vi "Comm_relay_sw..vi"(8 "Error in":errorcluster, 9 "Columns":i32[](array[numeric]), 10 "Row":i32, 11 "instrument handle in":refnum<k15>) -> (0 "error out":errorcluster, 3 "instrument handle out":refnum<k15>)   [LabVIEW 2016]
uses:
  <instrlib>/niSwitch/niSwitch.LLB/niSwitch Connect Channels (Single).vi
  <instrlib>/niSwitch/niSwitch.LLB/niSwitch Disconnect Channels (Single).vi
panel:
  in  "number of columns":i32=16
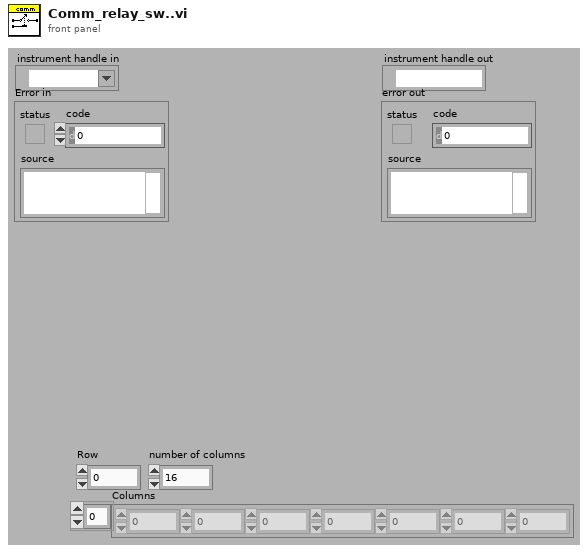
[diagram p1: front panel]
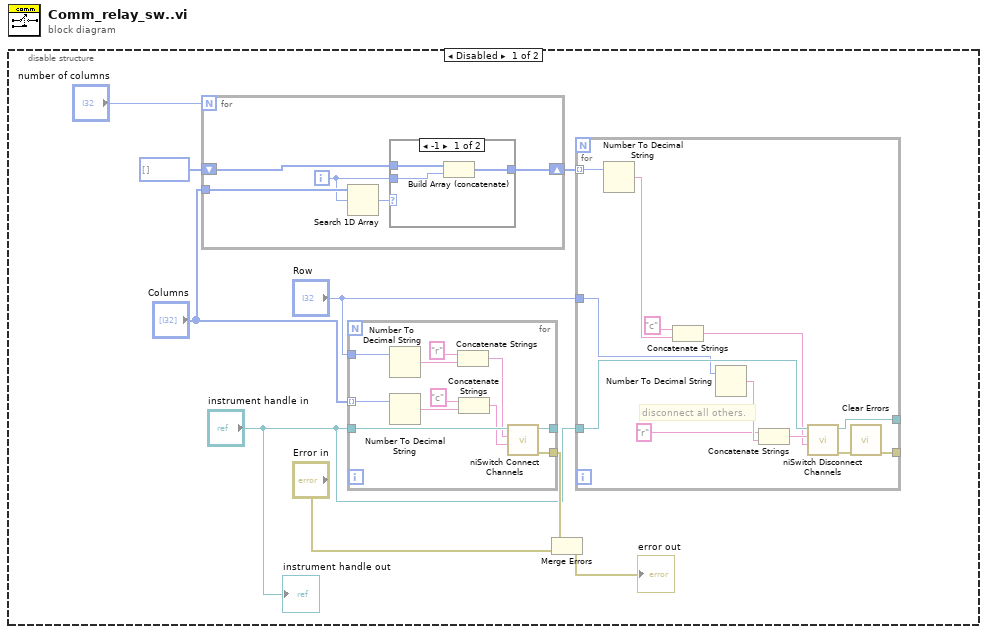
[diagram p0: block diagram]
diagram:
  n1 = disable-structure shown="Disabled" {
    frame Disabled {
      n2 = for {
        N: "number of columns" -> [_]
        tunnel: "Columns" -> [w26]
        shift-right: [w24] -> w6
        shift-left: i32[] [] -> [w23]
        i -> [w22]
        n3 = Search 1D Array(1D array=w26, element=w22) -> (index of element=w25:i32)  [unwired: 1 in]
        n4 = case shown="-1" w25 {
          tunnel: [w29 w30] -> w24
          tunnel: w23 -> [w28 w30]
          tunnel: w22 -> [w27 _]
          frame -1 {
            n5 = Build Array (concatenate)(w28, w27) -> (w29:i32[])
          }
          frame 0.., Default {
          }
        }
      }
      n6 = for {
        tunnel: "instrument handle in" -> [w41]
        tunnel: [w36] -> _
        tunnel: [w35] -> w4
        tunnel: "Columns" -> [w33] mode=indexing
        tunnel: "Row" -> [w32]
        n7 = Number To Decimal String(number=w32) -> (decimal integer string=w34:string)  [unwired: 1 in]
        n8 = Number To Decimal String(number=w33) -> (decimal integer string=w31:string)  [unwired: 1 in]
        n9 = Concatenate Strings("r" ("string"), w34) -> (w38:string)
        n10 = Concatenate Strings("c" ("string"), w31) -> (w37:string)
        n11 = call-poly <instrlib>:"niSwitch Connect Channels.vi"("channel 2"=w37, "channel 1"=w38, "instrument handle"=w41) -> ("error out"=w35:errorcluster, "instrument handle out"=w36:refnum<k15>)  [unwired: 7 in]
      }
      n12 = Merge Errors(w4, "Error in") -> (→"error out":errorcluster)
      n13 = for {
        tunnel: w6 -> [w14] mode=indexing
        tunnel: "instrument handle in" -> [w21]
        tunnel: [w20] -> _
        tunnel: [w10] -> _
        tunnel: "Row" -> [w13]
        # "disconnect all others."
        n14 = Number To Decimal String(number=w14) -> (decimal integer string=w18:string)  [unwired: 1 in]
        n15 = Concatenate Strings("c" ("string"), w18) -> (w11:string)
        n16 = Number To Decimal String(number=w13) -> (decimal integer string=w17:string)  [unwired: 1 in]
        n17 = Concatenate Strings("r" ("string"), w17) -> (w12:string)
        n18 = call-poly <instrlib>:"niSwitch Disconnect Channels.vi"("channel 2"=w11, "channel 1"=w12, "instrument handle"=w21) -> ("error out"=w19:errorcluster, "instrument handle out"=w20:refnum<k15>)  [unwired: 7 in]
        n19 = call <vilib>:"Clear Errors.vi"("error in (no error)"=w19) -> ("error out"=w10:errorcluster)  [unwired: 5 in, 1 out]
      }
      "instrument handle out" <- "instrument handle in"
    }
    frame Enabled {
    }
  }
